vi "MRT.vi"(0 "System no.":i32=1 min=1 max=4 step=1, 2 "Axes to move":string[](array[string]), 3 "Position values":dbl[](array[numeric]) format="%.6f", 4 "No.of digits":i16=4, 5 "error in":errorcluster) -> (19 "error out":errorcluster)   [LabVIEW 2026]
doc: "Executes a relative move in the tool coordinate system. No. of digits is the number of digits after the decimal point in the position value(s) that will be sent.\nTarget position results from calculating the translation first and then the rotation. Only hexapod axes can be moved. If no tool coordinate system is explicitly defined, the default tool coordinate system (0, 0, 0, 0, 0, 0) is used.\n\nC-887, F-206, M-8X0: Only for GCS syntax version = GCS 2.0 or higher (Check with CSV?.vi. If CSV?.vi is not supported, syntax version is GCS 1.0)."
panel:
  # "Executes a relative move in the Tool coordinate system."
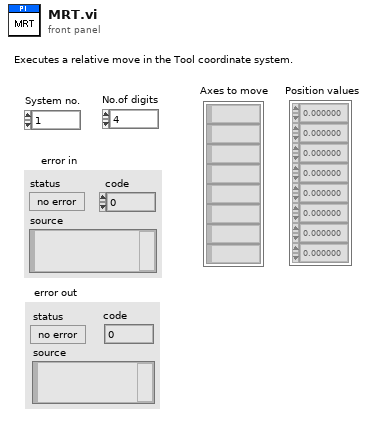
[diagram p1: front panel]
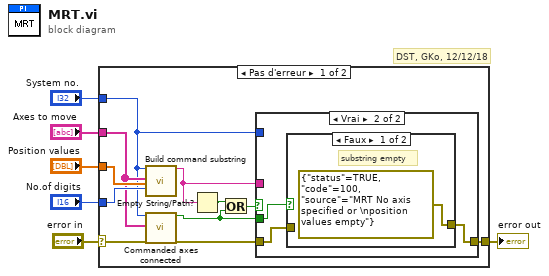
[diagram p0: block diagram]
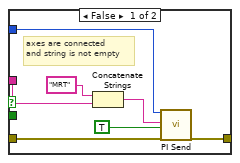
[diagram p2: hidden frame]
diagram:
  # "DST, GKo, 12/12/18"
  n1 = case shown="Pas d'erreur" "error in" {
    selector: "error in" -> [w10 w30]
    tunnel: [w17 w30] -> w6
    tunnel: "Position values" -> [w16 _]
    tunnel: "No.of digits" -> [w15 _]
    tunnel: "System no." -> [w11 _]
    tunnel: "Axes to move" -> [w13 _]
    frame No Error {
      n2 = call "Build command substring.vi"("System no."=w11, "Affected axes"=w13, "Parameters"=w16, "No. of digits"=w15) -> ("Command substring"=w9:string)  [unwired: 3 in, 12 out]
      n3 = call "Commanded axes connected.vi"("System no."=w11, "Commanded axes"=w13, "error in"=w10) -> ("Controller error"=w7:bool, "error out"=w14:errorcluster)  [unwired: 1 in, 14 out]
      n4 = Empty String/Path?(string/path=w9) -> (empty?=w8:bool)
      n5 = Or(x=w8, y=w7) -> (x .or. y?=w12:bool)
      n6 = case shown="Vrai" w12 {
        tunnel: w9 -> [w23 _]
        tunnel: [w19 w27] -> w17
        tunnel: w14 -> [w20 w26]
        tunnel: w11 -> [w18 _]
        tunnel: w7 -> [_ w25]
        frame False {
          # "axes are connected \nand string is not empty"
          n7 = Concatenate Strings("MRT", w23) -> (w21:string)
          n8 = call "PI Send.vi"("System no."=w18, "String to send"=w21, "Attach termination char.?"=TRUE ("Attach Linefeed?"), "error in"=w20) -> ("error out"=w19:errorcluster)  [unwired: 2 in, 13 out]
        }
        frame True {
          # "substring empty or axis not connected"
          n9 = case shown="Faux" w25 {
            tunnel: [errorcluster {"status"=TRUE, "code"=100, "source"="MRT No axis specified or \nposition values empty"} ("error out") w29] -> w27
            tunnel: w26 -> [_ w29]
            frame False {
              # "substring empty"
            }
            frame True {
              # "commanded axis not connected"
            }
          }
        }
      }
    }
    frame Error {
    }
  }
  "error out" <- w6
